vi "gui_T1.vi"(10 "input_xyz":T1) -> ()   [LabVIEW 2018]
uses:
  <vilib>/Analysis/NI_AALBase.lvlib
panel:
  in  "recenter_period_s":u32=5
  in  "recenter":bool=TRUE
  in  "show_all":bool
  in  "hide_all":bool
  out "elapsed_time_HMS":string
  in  "initial parameters":dbl[](array[numeric])=[0.5, 0.0001, 2.0, 100.0]
  out "estimated_time_HMS":string
  in  "plot_pulses":bool
  in  "gates_calculation":enum16{"Software", "Hardware"}(ring)=enum."Hardware"
  out "pulses":u32[][](graph)
  out "detections":u32[](graph)
  out "std. dev.":dbl format="%.3f"
  out "mean":dbl format="%0.2f"
  in  "auto_normalize":bool
  in  "normalize":bool
  in  "normalization_value":dbl=1.0 caption="Normalization value:" min=1.0 step=1.0
  out "status":string
  in  "use_proposed_width":bool
  in  "calc_width":bool
  in  "start":bool caption="Start"
  in  "save_file":bool
  out "contrast":dbl caption="Contrast :" format="%#_3f"
  in  "show_photons":bool
  in  "show_flags":bool
  out "mse":cluster{"read_widths_us":dbl[], "mse":dbl[]}(graph)
  in  "use_proposed_correction":bool
  out "proposed_read_width_us":dbl
  out "proposed_correction_us":dbl
  out "histogram":cluster{"histogram":i32[], "q_photons":i32[]}(graph)
  out "file_name":string caption="File name :"
  in  "sampling_mode":enum16{"Normal", "Sweep"}(ring)=enum."Sweep"
  out "quality":bool
  out "mse":dbl caption="Mean Square Error" format="%#.2e"
  out "T1_us":dbl format="%#.3g"
  out "T1 curves":cluster{dbl[], "dark_time_us":dbl[]}[](graph)
  in  "correction_us":dbl=0.65 caption="Delay"
  out "stop_count_photon":u32(colorbox)=16776704 caption="Stop Count & photon"
  out "stop_count":u32(colorbox)=6618880 caption="Stop Count"
  out "start_count_photon":u32(colorbox)=14417925 caption="Start Count & photon"
  out "start_count":u32(colorbox)=255 caption="Start Count"
  out "photon":u32(colorbox)=16448250 caption="Photon"
  out "noPhoton":u32(colorbox) caption="No Photon"
  out "photons_chart":u32[][](graph)
  in  "load_file":bool
  in  "refit":bool
  in  "read_width_us":dbl=1.0 caption="Width" min=0.0 max=10000.0 format="%#.3f"
  in  "read_delay_us":dbl caption="Delay"
  out "min_step":dbl format="%#.3f"
  in  "q_samples":i32=50
  in  "dt_stop_us":dbl=10000.0
  in  "dt_start_us":dbl=0.2
  in  "stop":bool
  in  "repetitions":i32=10000 caption="Repetitions" min=1 step=1
  in  "pulse_width_us":dbl=5.0 caption="Pulse width"
  # "Dark time [us]"
  # "*"
  # "*"
  # "us"
  # "*read_width_us and correction_us have to be multiple of 10ns\n*** start and stop markers are inside the detection gate. [start, stop]"
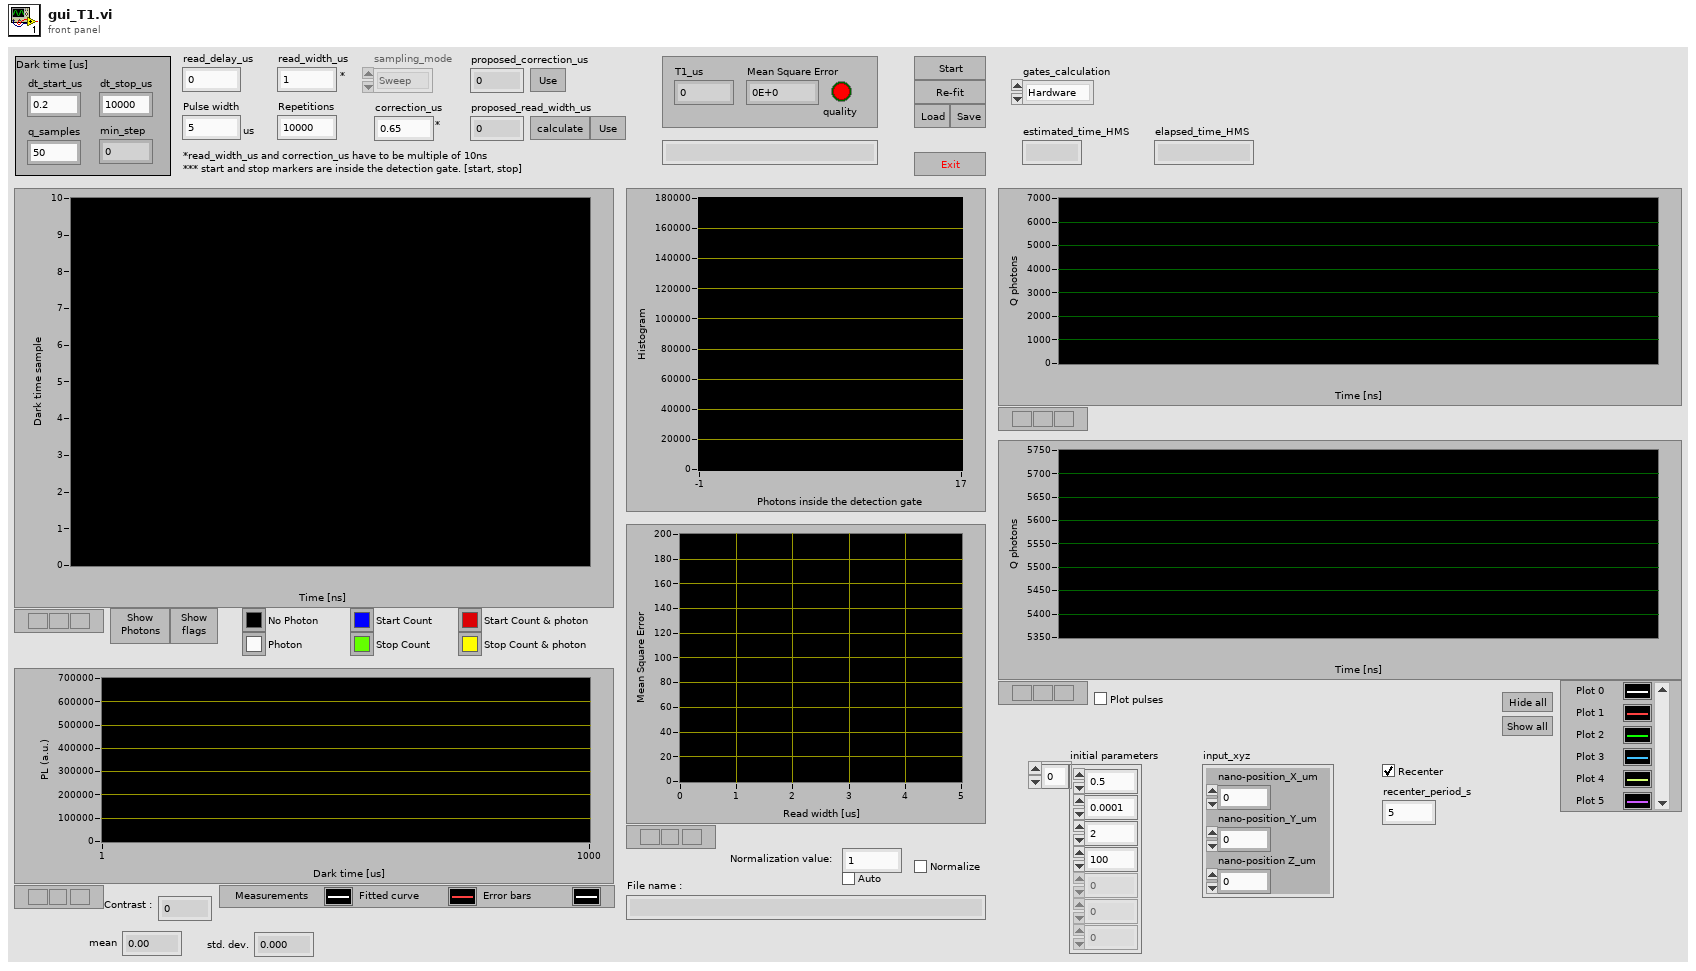
[diagram p1: front panel]
types:
  T1 = cluster{"nano-position_X_um":sgl, "nano-position_Y_um":sgl, "nano-position Z_um":sgl}
  T2 = cluster{"file_path":path, "file_name":string, "image":dbl[][][], "image_size_xy":cluster{"image_size_x_um":sgl, "image_size_y_um":sgl}, "pixel_dwell_time_ms":sgl, "Laser_power_mW":sgl, "pixel_size":dbl, "tile_ij":cluster{"tile_i":i32, "tile_j":i32}, "Objective":string, "ColorMarkers":cluster{dbl, u32}[], "timestamp":timestamp, "micro-position-xyz":cluster{"micro-position_x_mm":sgl, "micro-position_y_mm":sgl, "micro-position_z_mm":sgl}, "zero_xyz":cluster{"zero_x_mm":dbl, "zero_y_mm":dbl, "zero_z_mm":dbl}, "nano-position-xyz":cluster{"nano-position_x_V":sgl, "nano-position_y_V":sgl, "nano-position_z_V":sgl}, "Kxyz":cluster{"Kx_V/um":sgl, "Ky_V/um":sgl, "Kz_V/um":sgl}}
  T3 = cluster{"x_um":sgl[], "y_um":sgl[], "z_um":sgl[], "timetag":timestamp[]}
  T4 = cluster{"sampling_times":dbl[], "fitted_signal":dbl[]}
  T5 = cluster{"Ie":dbl, "Cm":dbl, "Tm":dbl, "C1":dbl, "T1":dbl, "mse":dbl}
  T6 = cluster{"dark_times_us":dbl[], "pulse_width_us":dbl, "read_delay_us":dbl, "read_width_us":dbl, "repetitions":i32, "sampling_mode":enum16{"Normal", "Sweep"}, "correction_us":dbl}
  T7 = cluster{"input_xyz":cluster{"nano-position_X_um":sgl, "nano-position_Y_um":sgl, "nano-position Z_um":sgl}, "recenter":bool, "recenter_s":u32}
  T8 = enum16{"standby", "doT1", "abort", "save", "re-fit", "load", "refresh", "use_proposed", "calcWidth"}
  T9 = cluster{"dark_times":dbl[], "fitted_signal":dbl[]}
  T10 = cluster{"dark_times_us":dbl[], "measured_signal":dbl[]}
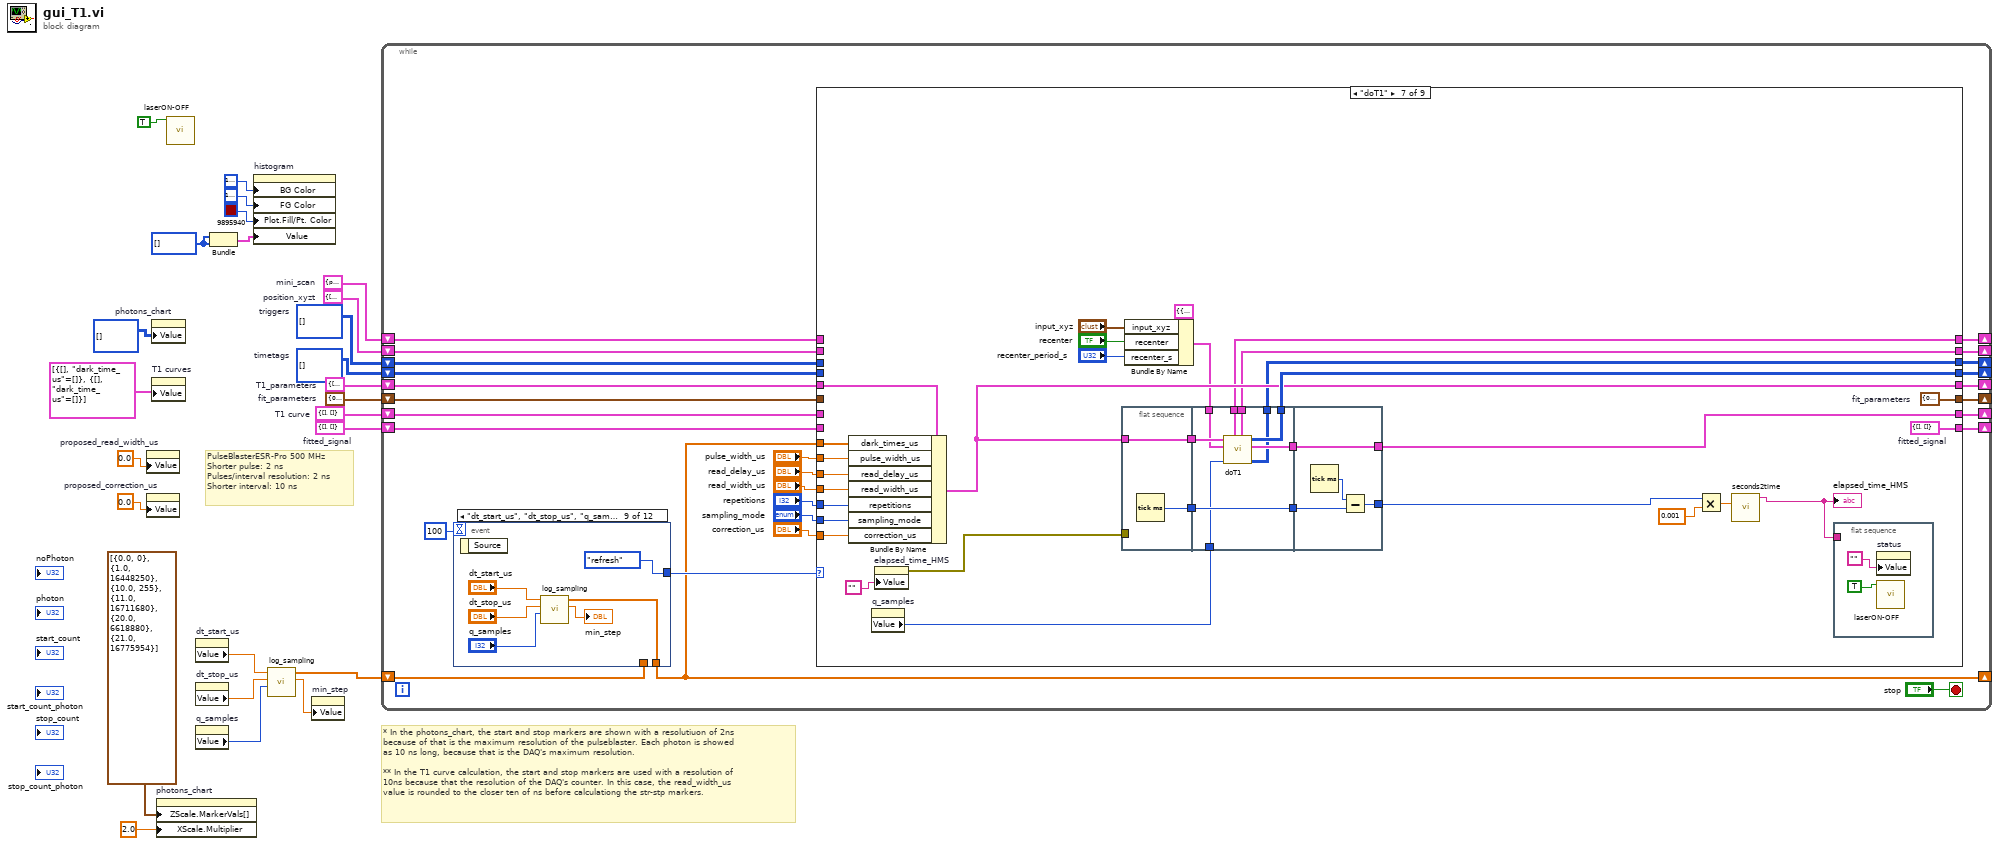
[diagram p0: block diagram]
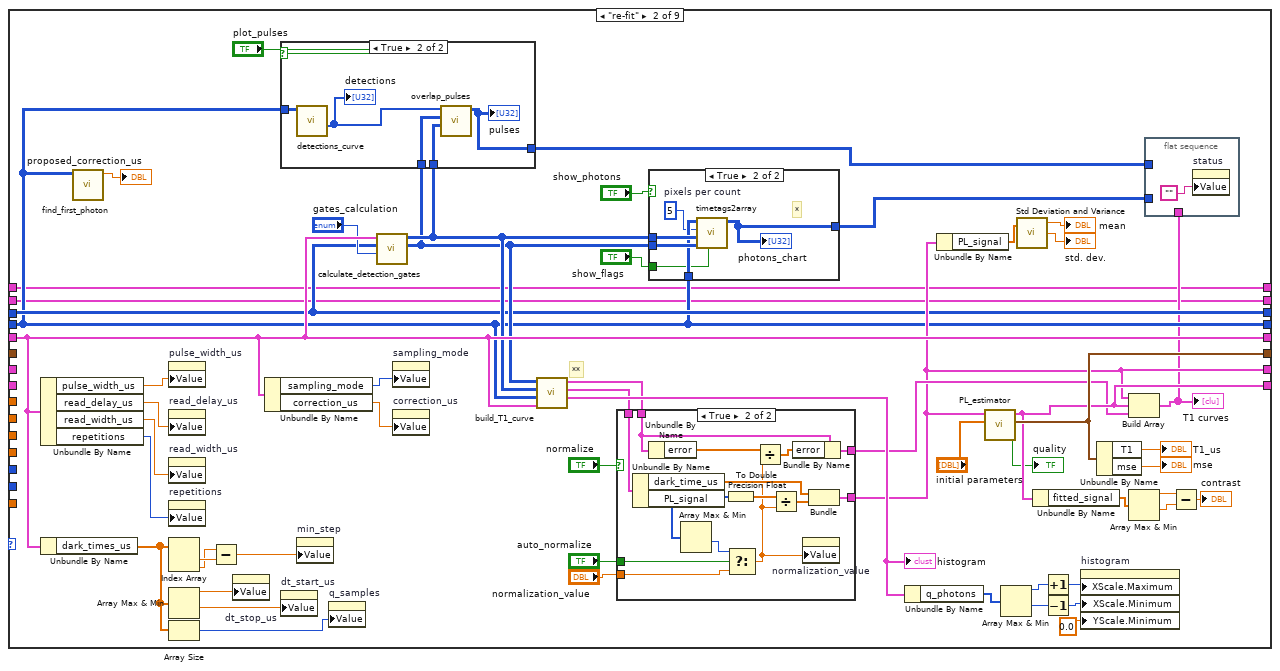
[diagram p3: hidden frame]
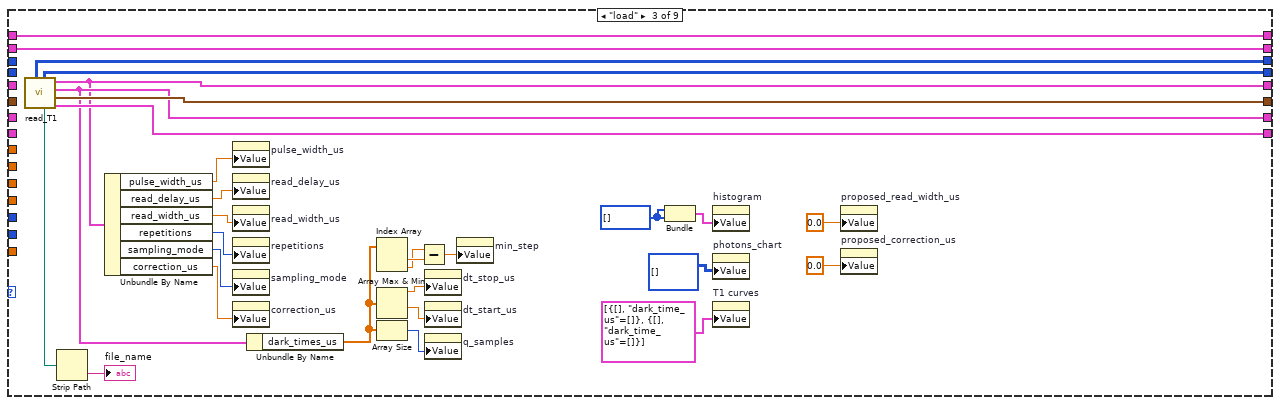
[diagram p7: hidden frame]
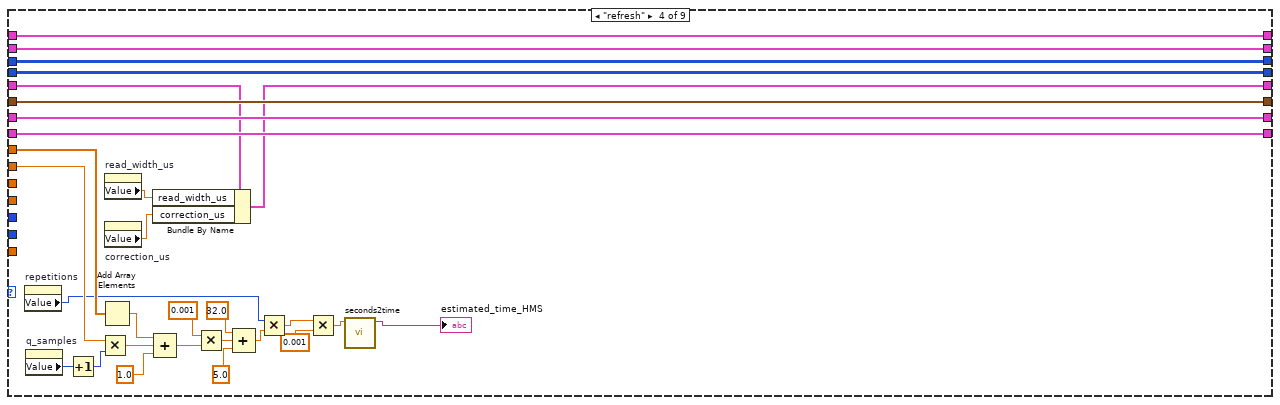
[diagram p8: hidden frame]
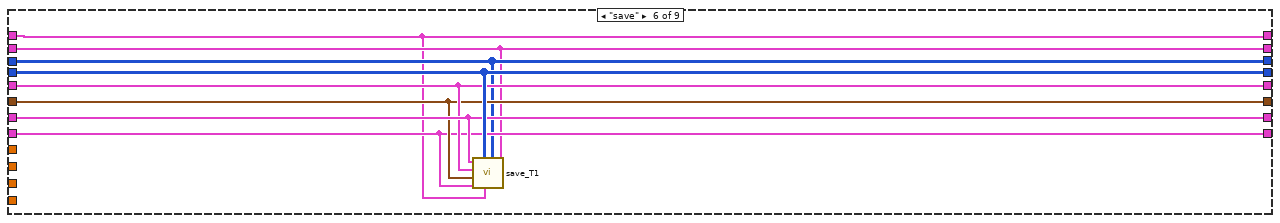
[diagram p10: hidden frame]
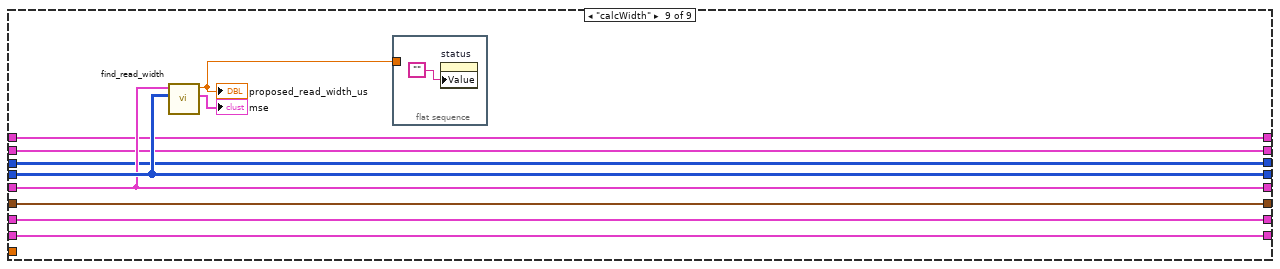
[diagram p12: hidden frame]
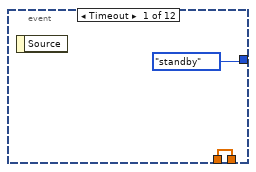
[diagram p13: hidden frame]
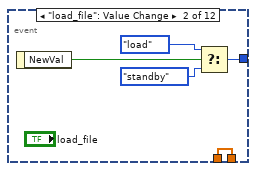
[diagram p14: hidden frame]
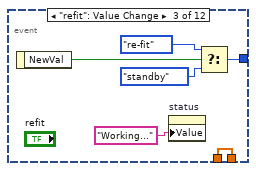
[diagram p15: hidden frame]
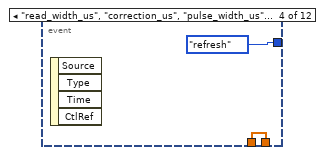
[diagram p16: hidden frame]
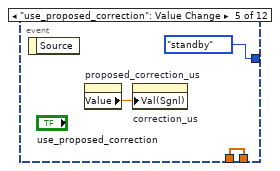
[diagram p17: hidden frame]
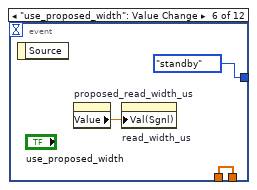
[diagram p18: hidden frame]
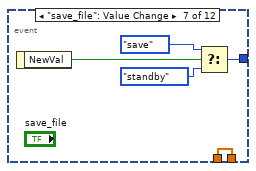
[diagram p19: hidden frame]
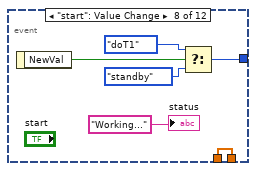
[diagram p20: hidden frame]
diagram:
  w1 = T2 {"file_path"=path "", "file_name"="", "image"=[], "image_size_xy"={"image_size_x_um"=0.0, "image_size_y_um"=0.0}, "pixel_dwell_time_ms"=0.0, "Laser_power_mW"=0.0, "pixel_size"=0.0, "tile_ij"={"tile_i"=0, "tile_j"=0}, "Objective"="", "ColorMarkers"=[], "timestamp"=timestamp(0 s since 1904-01-01), "micro-position-xyz"={"micro-position_x_mm"=0.0, "micro-position_y_mm"=0.0, "micro-position_z_mm"=0.0}, "zero_xyz"={"zero_x_mm"=0.0, "zero_y_mm"=0.0, "zero_z_mm"=0.0}, "nano-position-xyz"={"nano-position_x_V"=0.0, "nano-position_y_V"=0.0, "nano-position_z_V"=0.0}, "Kxyz"={"Kx_V/um"=0.0, "Ky_V/um"=0.0, "Kz_V/um"=0.0}}  # mini_scan
  w2 = T3 {"x_um"=[], "y_um"=[], "z_um"=[], "timetag"=[]}  # position_xyzt
  w4 = u32[][] []  # triggers
  w22 = T4 {"sampling_times"=[], "fitted_signal"=[]}  # fitted_signal
  w5 = u32[][] []  # timetags
  w23 = cluster{dbl[], "dark_time_us":dbl[]} {[], "dark_time_us"=[]}  # T1 curve
  w24 = T5 {"Ie"=0.0, "Cm"=0.0, "Tm"=0.0, "C1"=0.0, "T1"=0.0, "mse"=0.0}  # fit_parameters
  w21 = T6 {"dark_times_us"=[], "pulse_width_us"=0.0, "read_delay_us"=0.0, "read_width_us"=0.0, "repetitions"=0, "sampling_mode"=enum."Normal", "correction_us"=0.0}  # T1_parameters
  w16 = i32[] []
  # "* In the photons_chart, the start and stop markers are shown with a resolutiuon of 2ns \nbecause of that is the maximum resolution of the pulseblaster. Each photon is showed\nas 10 ns long, because that is the DAQ's maximum resolution.\n\n** In the T1 curve calculation, the start and stop markers are used with a resolution of\n10ns because that the resolution of the DAQ's counter. In this case, the read_width_us\nvalue is rounded to the closer ten of ns before calculationg the str-stp markers."
  # "PulseBlasterESR-Pro 500 MHz \nShorter pulse: 2 ns\nPulses/interval resolution: 2 ns\nShorter interval: 10 ns"
  n1 = property on="proposed_read_width_us" class="DigNum (strict)"("Value"=0.0 ("proposed_read_width_us")) -> ()  [unwired: 2 in, 2 out]
  n2 = property on="proposed_correction_us" class="DigNum (strict)"("Value"=0.0 ("proposed_correction_us")) -> ()  [unwired: 2 in, 2 out]
  n3 = property on="photons_chart" class="IntGraph (strict)"("Value"=i32[][] []) -> ()  [unwired: 2 in, 2 out]
  n4 = property on="T1 curves" class="XYGraph (strict)"("Value"=cluster{dbl[], "dark_time_us":dbl[]}[] [{[], "dark_time_us"=[]}, {[], "dark_time_us"=[]}] ("T1 curves")) -> ()  [unwired: 2 in, 2 out]
  n5 = property on="photons_chart" class="IntGraph (strict)"("ZScale.MarkerVals[]"=cluster{dbl, u32}[] [{0.0, 0}, {1.0, 16448250}, {10.0, 255}, {11.0, 16711680}, {20.0, 6618880}, {21.0, 16775954}] ("Z Scale.Marker Values[]"), "XScale.Multiplier"=2.0 ("X Scale.Offset and Multiplier:Multiplier")) -> ()  [unwired: 2 in, 2 out]
  n6 = call "laserON-OFF.vi"("ON-OFF"=TRUE) -> ()  [unwired: 11 in]
  n7 = property on="dt_start_us" class="DigNum (strict)"() -> ("Value"=w8:dbl)  [unwired: 2 in, 2 out]
  n8 = property on="dt_stop_us" class="DigNum (strict)"() -> ("Value"=w9:dbl)  [unwired: 2 in, 2 out]
  n9 = property on="q_samples" class="DigNum (strict)"() -> ("Value"=w10:i32)  [unwired: 2 in, 2 out]
  n10 = Bundle(w16, w16) -> (w15:cluster{i32[], i32[]})  [unwired: 1 in]
  n11 = property on="histogram" class="XYGraph (strict)"("BG Color"=u32 16777222 ("Plot Area:Colors:FG Color"), "FG Color"=u32 16777228 ("Plot Area:Colors:FG Color"), "Plot.Fill/Pt. Color"=u32 9895940 ("Plot Area:Colors:FG Color"), "Value"=w15) -> ()  [unwired: 2 in, 2 out]
  n12 = call "log_sampling.vi"("q_samples"=w10, "stop_us"=w9, "start_us"=w8) -> ("min_step_us"=w11:dbl, "sampling_times_us"=w7:dbl[])  [unwired: 7 in]
  n13 = property on="min_step" class="DigNum (strict)"("Value"=w11) -> ()  [unwired: 2 in, 2 out]
  n14 = while {
    shift-right: [w42] -> _
    shift-left: w21 -> [w49]
    shift-right: [w41] -> _
    shift-left: w24 -> [w48]
    shift-right: [w40] -> _
    shift-left: w23 -> [w47]
    shift-right: [w46] -> _
    shift-left: w22 -> [w45]
    shift-right: [w43] -> _
    shift-left: w5 -> [w44]
    shift-right: [w32] -> _
    shift-left: w7 -> [w33]
    shift-right: [w31] -> _
    shift-left: w4 -> [w30]
    shift-right: [w29] -> _
    shift-left: w2 -> [w28]
    shift-right: [w26] -> _
    shift-left: w1 -> [w27]
    stop <- "stop" stop-if-true
    n15 = event shown="[8] \"dt_start_us\", \"dt_stop_us\", \"q_samples\": Value Change" {
      selector: _ -> [_ _ _ _ _ _ _ _ _ _ _ _]
      dyn-events: _ -> [_ _ _ _ _ _ _ _ _ _ _ _]
      timeout: 100 -> [_ _ _ _ _ _ _ _ _ _ _ _]
      tunnel: [T8."standby" w291 w297 T8."refresh" T8."standby" T8."standby" w310 w317 T8."refresh" w329 T8."standby" T8."standby"] -> w50
      tunnel: w33 -> [w286 w288 w294 w299 w301 w304 w307 w312 _ w325 w332 w338]
      tunnel: [w286 w288 w294 w299 w301 w304 w307 w312 w319 w325 w332 w338] -> w32
      event Timeout {
        n16 = event-data() -> ()  [unwired: 1 in, 1 out]
      }
      event "load_file": Value Change {
        n17 = event-data() -> ("NewVal"=w292:bool)  [unwired: 1 in]
        n18 = Select(t=T8."load", s=w292, f=T8."standby") -> (s? t:f=w291:T8)
      }
      event "refit": Value Change {
        n19 = event-data() -> ("NewVal"=w298:bool)  [unwired: 1 in]
        n20 = property on="status" class="Str"("Value"="Working...") -> ()  [unwired: 2 in, 2 out]
        n21 = Select(t=T8."re-fit", s=w298, f=T8."standby") -> (s? t:f=w297:T8)
      }
      event "read_width_us", "correction_us", "pulse_width_us", "repetitions": Value Change {
        n22 = event-data() -> ()  [unwired: 1 in, 4 out]
      }
      event "use_proposed_correction": Value Change {
        n23 = event-data() -> ()  [unwired: 1 in, 1 out]
        n24 = property on="proposed_correction_us" class="DigNum (strict)"() -> ("Value"=w303:dbl)  [unwired: 2 in, 2 out]
        n25 = property on="correction_us" class="DigNum (strict)"("Val(Sgnl)"=w303) -> ()  [unwired: 2 in, 2 out]
      }
      event "use_proposed_width": Value Change {
        n26 = event-data() -> ()  [unwired: 1 in, 1 out]
        n27 = property on="proposed_read_width_us" class="DigNum (strict)"() -> ("Value"=w306:dbl)  [unwired: 2 in, 2 out]
        n28 = property on="read_width_us" class="DigNum (strict)"("Val(Sgnl)"=w306) -> ()  [unwired: 2 in, 2 out]
      }
      event "save_file": Value Change {
        n29 = event-data() -> ("NewVal"=w311:bool)  [unwired: 1 in]
        n30 = Select(t=T8."save", s=w311, f=T8."standby") -> (s? t:f=w310:T8)
      }
      event "start": Value Change {
        n31 = event-data() -> ("NewVal"=w316:bool)  [unwired: 1 in]
        n32 = Select(t=T8."doT1", s=w316, f=T8."standby") -> (s? t:f=w317:T8)
        "status" <- "Working..."
      }
      event "dt_start_us", "dt_stop_us", "q_samples": Value Change {
        n33 = event-data() -> ()  [unwired: 1 in, 1 out]
        n34 = call "log_sampling.vi"("q_samples"="q_samples", "stop_us"="dt_stop_us", "start_us"="dt_start_us") -> ("min_step_us"=→"min_step":dbl, "sampling_times_us"=w319:dbl[])  [unwired: 7 in]
      }
      event "calc_width": Value Change {
        n35 = event-data() -> ("NewVal"=w328:bool)  [unwired: 1 in]
        n36 = property on="status" class="Str"("Value"="Working...") -> ()  [unwired: 2 in, 2 out]
        n37 = Select(t=T8."calcWidth", s=w328, f=T8."standby") -> (s? t:f=w329:T8)
      }
      event "hide_all": Value Change {
        n38 = event-data() -> ()  [unwired: 1 in, 1 out]
        n39 = property on="q_samples" class="DigNum (strict)"() -> ("Value"=w330:i32)  [unwired: 2 in, 2 out]
        n40 = Increment(x=w330) -> (x+1=w331:i32)
        n41 = for {
          N: w331 -> [_]
          i -> [w335]
          n42 = property on="pulses" class="WFGraph (strict)"("Active Plot"=w335, "Plot.Visible?"=FALSE ("Plot.Visible")) -> ()  [unwired: 2 in, 2 out]
        }
      }
      event "show_all": Value Change {
        n43 = event-data() -> ()  [unwired: 1 in, 1 out]
        n44 = property on="q_samples" class="DigNum (strict)"() -> ("Value"=w336:i32)  [unwired: 2 in, 2 out]
        n45 = Increment(x=w336) -> (x+1=w337:i32)
        n46 = for {
          N: w337 -> [_]
          i -> [w341]
          n47 = property on="pulses" class="WFGraph (strict)"("Active Plot"=w341, "Plot.Visible?"=TRUE ("Plot.Visible")) -> ()  [unwired: 2 in, 2 out]
        }
      }
    }
    n48 = case shown="\"doT1\"" w50 {
      tunnel: w49 -> [w60 w92 _ w197 w208 w215 w249 w273 w282]
      tunnel: w48 -> [w59 _ _ w200 w207 w214 _ w272 w281]
      tunnel: w47 -> [w58 _ _ w199 w206 w216 _ w271 w280]
      tunnel: [w57 w89 w172 w198 w205 w213 w229 w270 w279] -> w46
      tunnel: w45 -> [w57 _ _ w198 w205 w213 _ w270 w279]
      tunnel: [w56 w66 w163 w201 w209 w217 w248 w274 w283] -> w43
      tunnel: w44 -> [w56 w66 _ w201 w209 w217 _ w274 w283]
      tunnel: [w60 w92 w165 w196 w208 w215 w239 w273 w282] -> w42
      tunnel: [w59 w115 w171 w200 w207 w214 w228 w272 w281] -> w41
      tunnel: [w58 w76 w170 w199 w206 w216 w240 w271 w280] -> w40
      tunnel: "read_delay_us" -> [_ _ _ _ _ _ w247 _ _]
      tunnel: "pulse_width_us" -> [_ _ _ w191 _ _ w246 _ _]
      tunnel: "read_width_us" -> [_ _ _ _ _ _ w245 _ _]
      tunnel: "repetitions" -> [_ _ _ _ _ _ w244 _ _]
      tunnel: "sampling_mode" -> [_ _ _ _ _ _ w243 _ _]
      tunnel: "correction_us" -> [_ _ _ _ _ _ w242 _ _]
      tunnel: w32 -> [_ _ _ w192 _ _ w241 _ _]
      tunnel: [w55 w67 w146 w193 w204 w212 w238 w269 w277] -> w31
      tunnel: w30 -> [w55 w67 _ w193 w204 w212 _ w269 w277]
      tunnel: [w54 w62 w145 w174 w203 w211 w222 w268 w276] -> w29
      tunnel: w28 -> [w54 w62 w145 w174 w203 w211 _ w268 w276]
      tunnel: [w53 w61 w144 w173 w202 w210 w219 w267 w275] -> w26
      tunnel: w27 -> [w53 w61 w144 w173 w202 w210 _ w267 w275]
      frame "standby", Default {
      }
      frame "re-fit" {
        # "**"
        n49 = Unbundle By Name(w92) -> ("pulse_width_us"=w107:dbl, "read_delay_us"=w106:dbl, "read_width_us"=w105:dbl, "repetitions"=w104:i32)
        n50 = Unbundle By Name(w92) -> ("dark_times_us"=w112:dbl[])
        n51 = call "find_first_photon.vi"("timetags"=w66) -> ("Numeric"=→"proposed_correction_us":dbl)  [unwired: 10 in]
        n52 = property on="pulse_width_us" class="DigNum (strict)"("Value"=w107) -> ()  [unwired: 2 in, 2 out]
        n53 = property on="read_delay_us" class="DigNum (strict)"("Value"=w106) -> ()  [unwired: 2 in, 2 out]
        n54 = property on="read_width_us" class="DigNum (strict)"("Value"=w105) -> ()  [unwired: 2 in, 2 out]
        n55 = property on="repetitions" class="DigNum (strict)"("Value"=w104) -> ()  [unwired: 2 in, 2 out]
        n56 = Index Array(array=w112) -> (element #1=w114:dbl, element #2=w113:dbl)  [unwired: 2 in]
        n57 = Array Max & Min(array=w112) -> (max value=w111:dbl, min value=w110:dbl)  [unwired: 2 out]
        n58 = Array Size(array=w112) -> (size(s)=w109:i32)
        n59 = Subtract(x=w113, y=w114) -> (x-y=w108:dbl)
        n60 = property on="dt_stop_us" class="DigNum (strict)"("Value"=w111) -> ()  [unwired: 2 in, 2 out]
        n61 = Unbundle By Name(w92) -> ("sampling_mode"=w102:enum16{"Normal", "Sweep"}, "correction_us"=w101:dbl)
        n62 = property on="dt_start_us" class="DigNum (strict)"("Value"=w110) -> ()  [unwired: 2 in, 2 out]
        n63 = property on="min_step" class="DigNum (strict)"("Value"=w108) -> ()  [unwired: 2 in, 2 out]
        n64 = property on="q_samples" class="DigNum (strict)"("Value"=w109) -> ()  [unwired: 2 in, 2 out]
        n65 = call "calculate_detection_gates.vi"("gates_calculation"="gates_calculation", "triggers"=w67, "T1_parameters"=w92) -> ("start_read"=w71:u32[][], "stop_read"=w72:u32[][])  [unwired: 7 in]
        n66 = case shown="True" "plot_pulses" {
          tunnel: w72 -> [_ w121]
          tunnel: w71 -> [_ w120]
          tunnel: w66 -> [_ w119]
          tunnel: [_ w117] -> w63
          frame False {
          }
          frame True {
            n67 = call "detections_curve.vi"("timetags"=w119) -> ("detections"=w118:u32[])  [unwired: 10 in]
            "detections" <- w118
            n68 = call "overlap_pulses.vi"("stop_read"=w121, "start_read"=w120, "detections"=w118) -> ("pulses"=w117:u32[][])  [unwired: 8 in]
            "pulses" <- w117
          }
        }
        n69 = property on="sampling_mode" class="Enum (strict)"("Value"=w102) -> ()  [unwired: 2 in, 2 out]
        n70 = property on="correction_us" class="DigNum (strict)"("Value"=w101) -> ()  [unwired: 2 in, 2 out]
        n71 = call "build_T1_curve.vi"("T1_parameters"=w92, "timetags"=w66, "stop_read"=w72, "start_read"=w71) -> ("histogram"=w100:cluster{"q_photons":i32[], "histogram":i32[]}, "T1 curve"=w70:cluster{"dark_time_us":dbl[], "PL_signal":i32[]}, "error_bars"=w79:cluster{"dark_times_us":dbl[], "error":dbl[]})  [unwired: 5 in]
        "histogram" <- w100
        n72 = case shown="True" "normalize" {
          tunnel: [w122 w137] -> w76
          tunnel: "normalization_value" -> [_ w128]
          tunnel: w79 -> [w123 w132]
          tunnel: [w123 w130] -> w78
          tunnel: "auto_normalize" -> [_ w126]
          tunnel: w70 -> [w122 w124]
          frame False {
          }
          frame True {
            n73 = Unbundle By Name(w124) -> ("dark_time_us"=w135:dbl[], "PL_signal"=w129:i32[])
            n74 = Unbundle By Name(w132) -> ("error"=w133:dbl[])
            n75 = Array Max & Min(array=w129) -> (min value=w127:i32)  [unwired: 3 out]
            n76 = To Double Precision Float(number=w129) -> (double precision float=w134:dbl[])
            n77 = Select(t=w127, s=w126, f=w128) -> (s? t:f=w125:dbl)
            n78 = Divide(x=w133, y=w125) -> (x/y=w131:dbl[])
            n79 = Divide(x=w134, y=w125) -> (x/y=w136:dbl[])
            n80 = Bundle By Name(cluster=w132, "error"=w131) -> (w130:cluster{"dark_times_us":dbl[], "error":dbl[]})
            n81 = property on="normalization_value" class="DigNum (strict)"("Value"=w125) -> ()  [unwired: 2 in, 2 out]
            n82 = Bundle("dark_time_us"=w135, w136) -> (w137:cluster{"dark_time_us":dbl[], dbl[]})  [unwired: 1 in]
          }
        }
        n83 = case shown="True" "show_photons" {
          tunnel: w71 -> [_ w143]
          tunnel: w72 -> [_ w142]
          tunnel: w66 -> [_ w141]
          tunnel: "show_flags" -> [_ w140]
          tunnel: [_ w138] -> w64
          frame False {
          }
          frame True {
            w139 = u32 5  # pixels per count
            # "*"
            n84 = call "timetags2array.vi"("show_flags"=w140, "start_read"=w143, "stop_read"=w142, "pixels/count"=w139, "timetags"=w141) -> ("photons_chart"=w138:u32[][])  [unwired: 6 in]
            "photons_chart" <- w138
          }
        }
        n85 = Unbundle By Name(w100) -> ("q_photons"=w99:i32[])
        n86 = Unbundle By Name(w76) -> ("PL_signal"=w75:dbl[])
        n87 = call "PL_estimator.vi"("initial parameters"="initial parameters", "measured_signal"=w76) -> ("quality_check"=→"quality":bool, "fit_parameters"=w115:T5, "fitted_signal"=w89:T4)  [unwired: 7 in]
        n88 = Array Max & Min(array=w99) -> (max value=w98:i32, min value=w96:i32)  [unwired: 2 out]
        n89 = call <vilib>:"Std Deviation and Variance.vi"("X"=w75) -> ("mean"=→"mean":dbl, "standard deviation"=→"std. dev.":dbl)  [unwired: 1 in, 1 out]
        n90 = Unbundle By Name(w89) -> ("fitted_signal"=w88:dbl[])
        n91 = Increment(x=w98) -> (x+1=w97:i32)
        n92 = Decrement(x=w96) -> (x-1=w95:i32)
        n93 = property on="histogram" class="XYGraph (strict)"("XScale.Maximum"=w97, "XScale.Minimum"=w95, "YScale.Minimum"=0.0 ("Y Scale.Range:Minimum")) -> ()  [unwired: 2 in, 2 out]
        n94 = Unbundle By Name(w115) -> ("T1"=→"T1_us":dbl, "mse"=→"mse":dbl)
        n95 = Build Array(w76, w89, w78) -> (w65:cluster{"dark_times_us":dbl[], "error":dbl[]}[])
        "T1 curves" <- w65
        n96 = Array Max & Min(array=w88) -> (max value=w87:dbl, min value=w86:dbl)  [unwired: 2 out]
        n97 = flat-sequence {
          tunnel: w65 -> [_]
          tunnel: w64 -> [_]
          tunnel: w63 -> [_]
          frame #0 {
            n98 = property on="status" class="Str"("Value"="") -> ()  [unwired: 2 in, 2 out]
          }
        }
        n99 = Subtract(x=w87, y=w86) -> (x-y=→"contrast":dbl)
      }
      frame "load" {
        w160 = i32[] []
        n100 = call "read_T1.vi"() -> ("fitted_signal"=w172:T9, "fit_parameters"=w171:T5, "T1_curve"=w170:T10, "T1_parameters"=w165:T6, "file_path"=w162:path, "timetags"=w163:u32[][], "triggers"=w146:u32[][])  [unwired: 5 in]
        n101 = Strip Path(path=w162) -> (name=→"file_name":string)  [unwired: 1 out]
        n102 = Unbundle By Name(w165) -> ("pulse_width_us"=w154:dbl, "read_delay_us"=w153:dbl, "read_width_us"=w166:dbl, "repetitions"=w151:i32, "sampling_mode"=w152:enum16{"Normal", "Sweep"}, "correction_us"=w164:dbl)
        n103 = property on="pulse_width_us" class="DigNum (strict)"("Value"=w154) -> ()  [unwired: 2 in, 2 out]
        n104 = property on="read_delay_us" class="DigNum (strict)"("Value"=w153) -> ()  [unwired: 2 in, 2 out]
        n105 = property on="read_width_us" class="DigNum (strict)"("Value"=w166) -> ()  [unwired: 2 in, 2 out]
        n106 = property on="repetitions" class="DigNum (strict)"("Value"=w151) -> ()  [unwired: 2 in, 2 out]
        n107 = property on="sampling_mode" class="Enum (strict)"("Value"=w152) -> ()  [unwired: 2 in, 2 out]
        n108 = property on="correction_us" class="DigNum (strict)"("Value"=w164) -> ()  [unwired: 2 in, 2 out]
        n109 = Unbundle By Name(w170) -> ("dark_times_us"=w169:dbl[])
        n110 = Index Array(array=w169) -> (element #1=w168:dbl, element #2=w167:dbl)  [unwired: 2 in]
        n111 = Array Max & Min(array=w169) -> (max value=w148:dbl, min value=w149:dbl)  [unwired: 2 out]
        n112 = Array Size(array=w169) -> (size(s)=w150:i32)
        n113 = Subtract(x=w167, y=w168) -> (x-y=w147:dbl)
        n114 = property on="dt_stop_us" class="DigNum (strict)"("Value"=w148) -> ()  [unwired: 2 in, 2 out]
        n115 = property on="dt_start_us" class="DigNum (strict)"("Value"=w149) -> ()  [unwired: 2 in, 2 out]
        n116 = property on="q_samples" class="DigNum (strict)"("Value"=w150) -> ()  [unwired: 2 in, 2 out]
        n117 = property on="min_step" class="DigNum (strict)"("Value"=w147) -> ()  [unwired: 2 in, 2 out]
        n118 = Bundle(w160, w160) -> (w159:cluster{i32[], i32[]})  [unwired: 1 in]
        n119 = property on="histogram" class="XYGraph (strict)"("Value"=w159) -> ()  [unwired: 2 in, 2 out]
        n120 = property on="photons_chart" class="IntGraph (strict)"("Value"=i32[][] []) -> ()  [unwired: 2 in, 2 out]
        n121 = property on="T1 curves" class="XYGraph (strict)"("Value"=cluster{dbl[], "dark_time_us":dbl[]}[] [{[], "dark_time_us"=[]}, {[], "dark_time_us"=[]}] ("T1 curves")) -> ()  [unwired: 2 in, 2 out]
        n122 = property on="proposed_read_width_us" class="DigNum (strict)"("Value"=0.0 ("proposed_read_width_us")) -> ()  [unwired: 2 in, 2 out]
        n123 = property on="proposed_correction_us" class="DigNum (strict)"("Value"=0.0 ("proposed_correction_us")) -> ()  [unwired: 2 in, 2 out]
      }
      frame "refresh" {
        n124 = property on="repetitions" class="DigNum (strict)"() -> ("Value"=w179:i32)  [unwired: 2 in, 2 out]
        n125 = property on="q_samples" class="DigNum (strict)"() -> ("Value"=w190:i32)  [unwired: 2 in, 2 out]
        n126 = Increment(x=w190) -> (x+1=w189:i32)
        n127 = Multiply(x=w191, y=w189) -> (x*y=w187:dbl)
        n128 = Add Array Elements(numeric array=w192) -> (sum=w188:dbl)
        n129 = property on="read_width_us" class="DigNum (strict)"() -> ("Value"=w195:dbl)  [unwired: 2 in, 2 out]
        n130 = property on="correction_us" class="DigNum (strict)"() -> ("Value"=w194:dbl)  [unwired: 2 in, 2 out]
        n131 = Bundle By Name(cluster=w197, "read_width_us"=w195, "correction_us"=w194) -> (w196:T6)
        n132 = Compound Arithmetic op=ADD(w188, w187, 1.0 ("value")) -> (w185:dbl)
        n133 = Multiply(x=0.001, y=w185) -> (x*y=w183:dbl)
        n134 = Compound Arithmetic op=ADD(32.0 ("value"), w183, 5.0 ("value")) -> (w180:dbl)
        n135 = Multiply(x=w179, y=w180) -> (x*y=w178:dbl)
        n136 = Multiply(x=w178, y=0.001 ("x")) -> (x*y=w176:dbl)
        n137 = call "seconds2time.vi"("seconds"=w176) -> ("HH:MM:SS"=→"estimated_time_HMS":string)  [unwired: 10 in]
      }
      frame "use_proposed" {
      }
      frame "save" {
        n138 = call "save_T1.vi"("position_xyzt"=w211, "triggers"=w212, "image_info"=w210, "timetags"=w217, "fitted_signal_in"=w213, "fit_parameters"=w214, "T1_parameters"=w215, "T1_curve_in"=w216) -> ()  [unwired: 4 in]
      }
      frame "doT1" {
        w228 = T5 {"Ie"=0.0, "Cm"=0.0, "Tm"=0.0, "C1"=0.0, "T1"=0.0, "mse"=0.0}  # fit_parameters
        w229 = T4 {"sampling_times"=[], "fitted_signal"=[]}  # fitted_signal
        n139 = Bundle By Name(cluster=w249, "dark_times_us"=w241, "pulse_width_us"=w246, "read_delay_us"=w247, "read_width_us"=w245, "repetitions"=w244, "sampling_mode"=w243, "correction_us"=w242) -> (w239:T6)
        n140 = property on="q_samples" class="DigNum (strict)"() -> ("Value"=w218:i32)  [unwired: 2 in, 2 out]
        n141 = property on="elapsed_time_HMS" class="Str"("Value"="") -> (error out=w231:errorcluster)  [unwired: 2 in, 1 out]
        n142 = flat-sequence {
          tunnel: w239 -> [w251]
          tunnel: [w251] -> w237
          tunnel: [w250] -> w234
          tunnel: w231 -> [_]
          tunnel: [w260] -> w248
          tunnel: [w257] -> w238
          tunnel: w237 -> [w258]
          tunnel: [w259] -> w236
          tunnel: [w256] -> w235
          tunnel: w234 -> [w256]
          tunnel: w225 -> [w255]
          tunnel: [w254] -> w222
          tunnel: [w253] -> w219
          tunnel: w218 -> [w252]
          tunnel: [w264] -> w240
          tunnel: w236 -> [w264]
          tunnel: w235 -> [w262]
          tunnel: [w261] -> w226
          frame #0 {
            n143 = Tick Count (ms)() -> (millisecond timer value=w250:u32)
          }
          frame #1 {
            n144 = call "doT1.vi"("q_samples"=w252, "parameters_recenter"=w255, "Rabi_parameters"=w258) -> ("triggers"=w257:u32[][], "Rabi_curve"=w259:cluster{dbl[], "dark_time_us":dbl[]}, "timetags"=w260:u32[][], "position_xyzt"=w254:T3, "mini_scan"=w253:T2)  [unwired: 3 in, 1 out]
          }
          frame #2 {
            n145 = Tick Count (ms)() -> (millisecond timer value=w263:u32)
            n146 = Subtract(x=w263, y=w262) -> (x-y=w261:u32)
          }
        }
        n147 = Bundle By Name(cluster=T7 {"input_xyz"={"nano-position_X_um"=0.0, "nano-position_Y_um"=0.0, "nano-position Z_um"=0.0}, "recenter"=FALSE, "recenter_s"=3} ("parameters_recenter"), "input_xyz"="input_xyz", "recenter"="recenter", "recenter_s"="recenter_period_s") -> (w225:T7)
        n148 = Multiply(x=w226, y=0.001) -> (x*y=w233:dbl)
        n149 = call "seconds2time.vi"("seconds"=w233) -> ("HH:MM:SS"=w227:string)  [unwired: 10 in]
        "elapsed_time_HMS" <- w227
        n150 = flat-sequence {
          tunnel: w227 -> [_]
          frame #0 {
            n151 = property on="status" class="Str"("Value"="") -> ()  [unwired: 2 in, 2 out]
            n152 = call "laserON-OFF.vi"("ON-OFF"=TRUE) -> ()  [unwired: 11 in]
          }
        }
      }
      frame "abort" {
      }
      frame "calcWidth" {
        n153 = call "find_read_width.vi"("timetags"=w283, "T1_parameters"=w282) -> ("mse"=→"mse":cluster{"read_widths_us":dbl[], "mse":dbl[]}, "proposed_read_width_us"=w278:dbl)  [unwired: 8 in]
        "proposed_read_width_us" <- w278
        n154 = flat-sequence {
          tunnel: w278 -> [_]
          frame #0 {
            n155 = property on="status" class="Str"("Value"="") -> ()  [unwired: 2 in, 2 out]
          }
        }
      }
    }
  }
